vi "Config Chans Clock and Start Scanning.vi"(4 "bypass":bool, 5 "Rate":dbl=10000.0 caption="Sample Rate (Hz)" format="%0.2f", 6 "stop&start now?":bool, 7 "sample mode":i32(ring)=10178 items=["Finite Samples"=10178, "Continuous Samples"=10123], 8 "error_in":errorcluster, 10 "SamplesPerChan":i32=1000 caption="Samples per Channel", 11 "Task in":refnum<k21>) -> (0 "error_out":errorcluster, 3 "task out":refnum<k21>)   [LabVIEW 2017, in "DAQ.lvclass"]
doc: "Developed by Kevin Thompson\nThompson Engineering, LLC\nkevin@thompsonengineering.net"
uses:
  DAQ.lvclass
  <vilib>/DAQmx/configure/timing.llb/DAQmx Timing (Sample Clock).vi
panel:
  # "Note: SamplesPerChan required if\nsample mode = \"Finite Samples\""
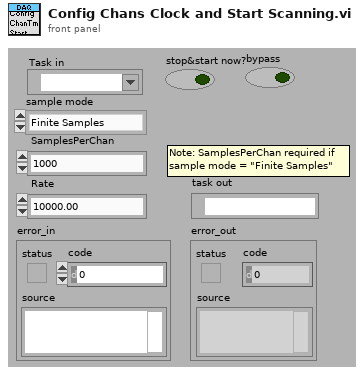
[diagram p1: front panel]
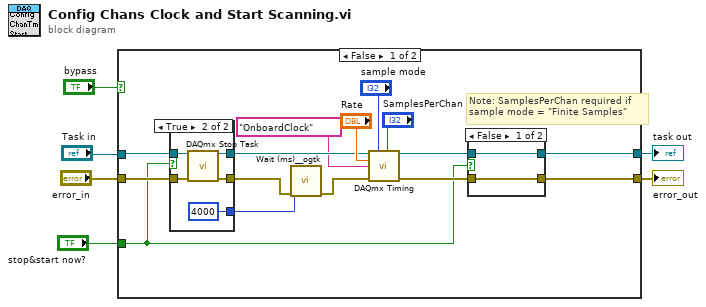
[diagram p0: block diagram]
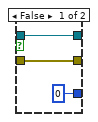
[diagram p2: hidden frame]
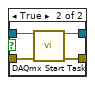
[diagram p3: hidden frame]
diagram:
  n1 = case shown="False" "bypass" {
    tunnel: [w16 w36] -> w6
    tunnel: [w15 w37] -> w5
    tunnel: "error_in" -> [w14 w36]
    tunnel: "Task in" -> [w12 w37]
    tunnel: "stop&start now?" -> [w8 _]
    frame False {
      # "Note: SamplesPerChan required if\nsample mode = \"Finite Samples\""
      n2 = case shown="True" w8 {
        tunnel: w14 -> [w23 w29]
        tunnel: [w24 w28] -> w13
        tunnel: w12 -> [w24 w27]
        tunnel: [w23 w26] -> w11
        tunnel: [u32 0 ("wait (ms)") u32 4000 ("wait (ms)")] -> w7
        frame False {
        }
        frame True {
          n3 = call <vilib>:"DAQmx Stop Task.vi"("task/channels in"=w27, "error in"=w29) -> ("task out"=w28:refnum<k21>, "error out"=w26:errorcluster)  [unwired: 12 in]
        }
      }
      n4 = call <userlib>:"Wait (ms)__ogtk.vi"("error in (no error)"=w11, "milliseconds to wait"=w7) -> ("error out"=w10:errorcluster)  [unwired: 8 in, 1 out]
      n5 = call-poly <vilib>:"DAQmx Timing.vi"("task/channels in"=w13, "sample mode"="sample mode", "samples per channel"="SamplesPerChan", "rate"="Rate", "source"=tag "OnboardClock", "error in"=w10) -> ("task out"=w17:refnum<k21>, "error out"=w18:errorcluster)  [unwired: 8 in]
      n6 = case shown="False" w8 {
        tunnel: w18 -> [w30 w35]
        tunnel: w17 -> [w31 w34]
        tunnel: [w30 w33] -> w16
        tunnel: [w31 w32] -> w15
        frame False {
        }
        frame True {
          n7 = call <vilib>:"DAQmx Start Task.vi"("task/channels in"=w34, "error in"=w35) -> ("task out"=w32:refnum<k21>, "error out"=w33:errorcluster)  [unwired: 12 in]
        }
      }
    }
    frame True {
    }
  }
  "error_out" <- w6
  "task out" <- w5
